vi "Execute RPC.vi"(6 "timeout (s)":dbl=60.0 format="%#_13g", 7 "encrypt (false)":bool, 8 "error in (no error)":errorcluster, 9 "request":u8[](array[numeric]), 10 "RPC Command":T1 items=["Debug Print", "Configure ATECC", "Set Signed Identity", "Erase Bonds and Power Off", "Get Spider Cal Constants", "Get Reset Reason", "Get Fault Log", "Set Mac Address"], 11 "target endpoint MAC address in":string="fd:e1:33:41:58:d3") -> (0 "error out":errorcluster, 2 "response":u8[](array[numeric]), 3 "target endpoint MAC address out":string)   [LabVIEW 2017]
uses:
  <vilib>/addons/InsightCM/Utilities/BleBackdoor/RPC Commands.ctl
  <vilib>/ErrorRing/Error Ring.xnode
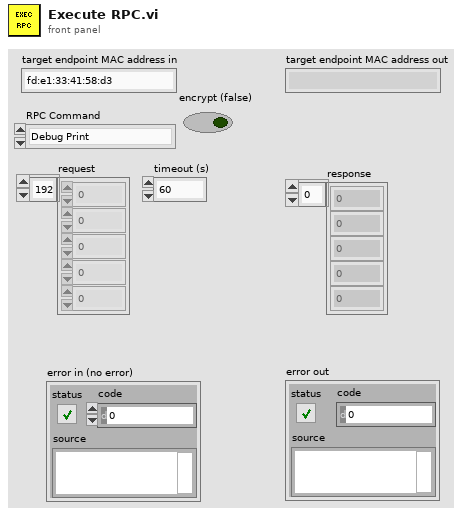
[diagram p1: front panel]
types:
  T1 = typedef "RPC Commands.ctl" = u16
  T2 = cluster{"[0]":u8, "[1]":u8, "[2]":u8, "[3]":u8, "[4]":u8, "[5]":u8, "[6]":u8, "[7]":u8, "[8]":u8}
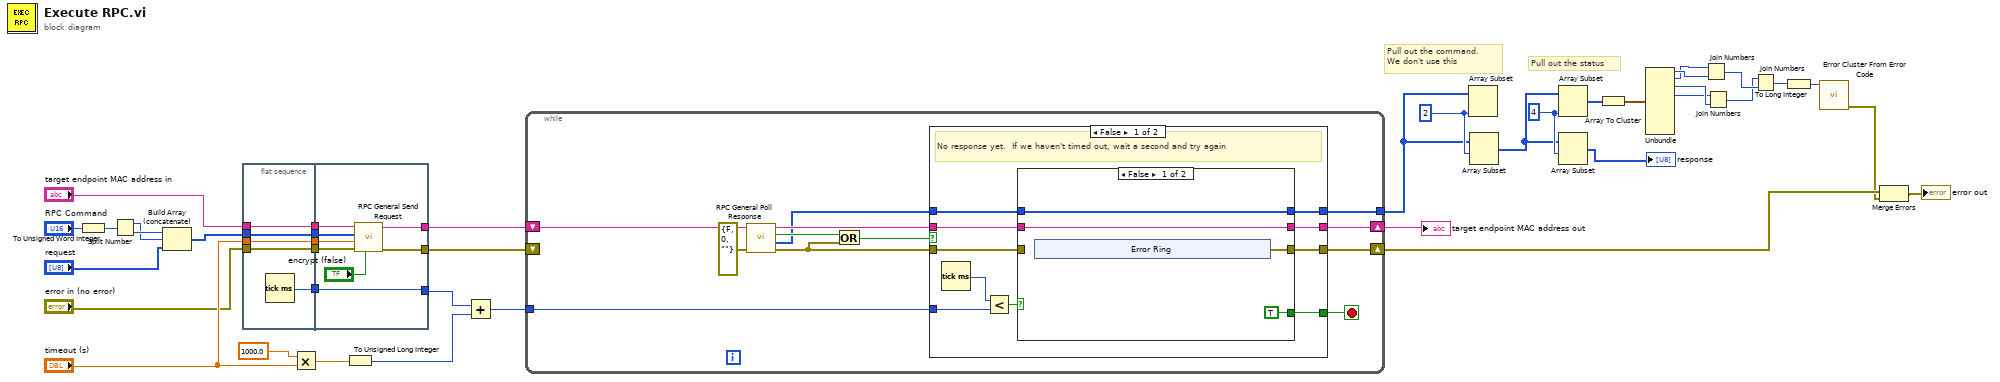
[diagram p0: block diagram]
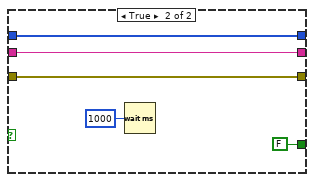
[diagram p2: hidden frame]
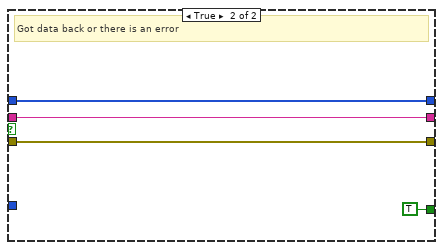
[diagram p3: hidden frame]
diagram:
  w16 = 4 ("length")
  w18 = 2 ("length")
  # "Pull out the status"
  # "Pull out the command.\nWe don't use this"
  n1 = To Unsigned Word Integer(number="RPC Command") -> (unsigned 16bit integer=w38:T1)
  n2 = Split Number(x=w38) -> (hi(x)=w36:u8, lo(x)=w37:u8)
  n3 = Build Array (concatenate)(w37, w36, "request") -> (w34:u8[])
  n4 = flat-sequence {
    tunnel: "timeout (s)" -> [w43]
    tunnel: w34 -> [w44]
    tunnel: "target endpoint MAC address in" -> [w45]
    tunnel: [w45] -> w31
    tunnel: [w44] -> w30
    tunnel: [w43] -> w29
    tunnel: [w42] -> w28
    tunnel: "error in (no error)" -> [w41]
    tunnel: [w41] -> w21
    tunnel: w31 -> [w53]
    tunnel: w30 -> [w52]
    tunnel: w29 -> [w51]
    tunnel: w28 -> [w48]
    tunnel: w21 -> [w47]
    tunnel: [w50] -> w33
    tunnel: [w49] -> w32
    tunnel: [w48] -> w27
    frame #0 {
      n5 = Tick Count (ms)() -> (millisecond timer value=w42:u32)
    }
    frame #1 {
      n6 = call <vilib>:"RPC General Send Request.vi"("encrypt (false)"="encrypt (false)", "error in (no error)"=w47, "time limit (60s)"=w51, "request"=w52, "BLE address in"=w53) -> ("error out"=w49:errorcluster, "BLE address out"=w50:string)  [unwired: 5 in]
    }
  }
  n7 = Multiply(x=1000.0, y="timeout (s)") -> (x*y=w24:dbl)
  n8 = To Unsigned Long Integer(number=w24) -> (unsigned 32bit integer=w23:u32)
  n9 = Add(x=w27, y=w23) -> (x+y=w22:u32)
  n10 = while {
    shift-right: [w62] -> w19
    shift-left: w33 -> [w65]
    shift-right: [w64] -> w11
    shift-left: w32 -> [_]
    tunnel: w22 -> [w58]
    tunnel: [w55] -> w17
    stop <- w57 stop-if-true
    n11 = call <vilib>:"RPC General Poll Response.vi"("error in (no error)"=errorcluster {"status"=FALSE, "code"=0, "source"=""}, "BLE address in"=w65) -> ("error out"=w59:errorcluster, "response"=w56:u8[], "polled"=w60:bool, "BLE address out"=w63:string)  [unwired: 6 in]
    n12 = Or(x=w60, y=w59) -> (x .or. y?=w61:bool)
    n13 = case shown="False" w61 {
      tunnel: w59 -> [w70 w92]
      tunnel: [w69 w92] -> w64
      tunnel: w63 -> [w72 w91]
      tunnel: [w71 w91] -> w62
      tunnel: w58 -> [w74 _]
      tunnel: [w68 TRUE] -> w57
      tunnel: w56 -> [w67 w89]
      tunnel: [w66 w89] -> w55
      frame False {
        # "No response yet.  If we haven't timed out, wait a second and try again"
        n14 = Tick Count (ms)() -> (millisecond timer value=w75:u32)
        n15 = Less?(x=w75, y=w74) -> (x < y?=w73:bool)
        n16 = case shown="False" w73 {
          tunnel: w72 -> [w79 w87]
          tunnel: [w79 w87] -> w71
          tunnel: w70 -> [_ w86]
          tunnel: [w78 w86] -> w69
          tunnel: [TRUE FALSE] -> w68
          tunnel: w67 -> [w76 w84]
          tunnel: [w76 w84] -> w66
          frame False {
            n17 = xnode "Error Ring"() -> ("error out"=w78:errorcluster)
          }
          frame True {
            n18 = Wait (ms)(milliseconds to wait=u32 1000) -> ()  [unwired: 1 out]
          }
        }
      }
      frame True {
        # "Got data back or there is an error"
      }
    }
  }
  "target endpoint MAC address out" <- w19
  n19 = Array Subset(array=w17, length=w18) -> ()  [unwired: 1 in, 1 out]
  n20 = Array Subset(array=w17, index=w18) -> (w15:u8[])  [unwired: 1 in]
  n21 = Array Subset(array=w15, length=w16) -> (w14:u8[])  [unwired: 1 in]
  n22 = Array Subset(array=w15, index=w16) -> (→"response":u8[])  [unwired: 1 in]
  n23 = Array To Cluster(array=w14) -> (cluster=w13:T2)
  n24 = Unbundle(w13) -> ("[0]"=w9:u8, "[1]"=w8:u8, "[2]"=w7:u8, "[3]"=w6:u8)  [unwired: 5 out]
  n25 = Join Numbers(hi=w8, lo=w9) -> ((hi.lo)=w5:u16)
  n26 = Join Numbers(hi=w6, lo=w7) -> ((hi.lo)=w4:u16)
  n27 = Join Numbers(hi=w4, lo=w5) -> ((hi.lo)=w12:u32)
  n28 = To Long Integer(number=w12) -> (32bit integer=w3:i32)
  n29 = call <vilib>:"Error Cluster From Error Code.vi"("error code (0)"=w3) -> ("error out"=w2:errorcluster)  [unwired: 8 in]
  n30 = Merge Errors(w11, w2) -> (→"error out":errorcluster)
